vi "Read Image Delays.vi"(8 "error in (no error)":errorcluster, 11 "Header Contents in":refnum<class "Header Contents.lvclass">) -> (0 "error out":errorcluster, 2 "Image Delays":string[](array[string]), 3 "Header Contents out":refnum<class "Header Contents.lvclass">)   [LabVIEW 2018, in "Header Contents.lvclass"]
uses:
  Header Contents.lvclass
  Header Contents.lvclass/Header Contents.ctl
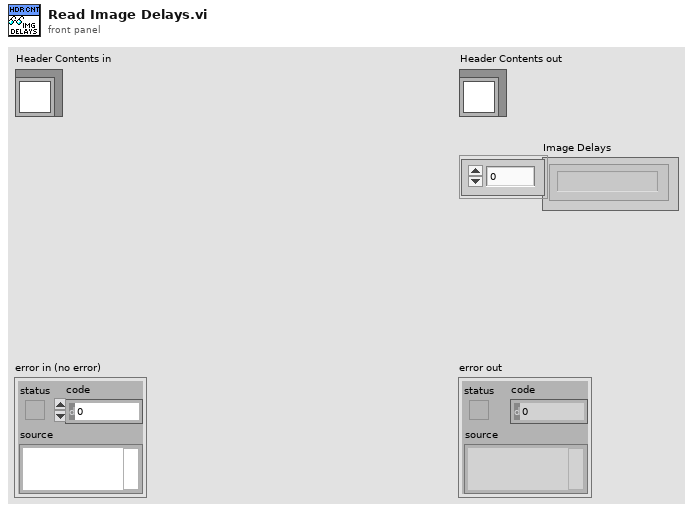
[diagram p1: front panel]
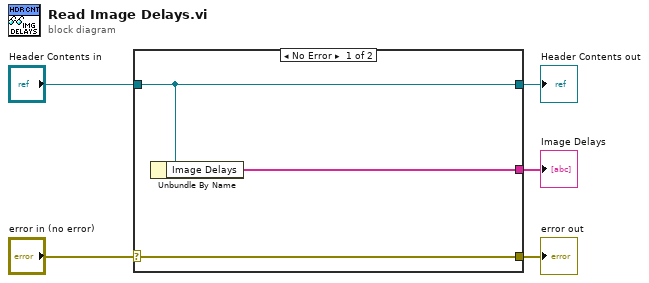
[diagram p0: block diagram]
diagram:
  n1 = case shown="No Error" "error in (no error)" {
    selector: "error in (no error)" -> [w8 w9]
    tunnel: [w8 w9] -> w4
    tunnel: [w7 w10] -> w2
    tunnel: "Header Contents in" -> [w7 w10]
    tunnel: [w6 _] -> w1
    frame No Error {
      n2 = Unbundle By Name(w7) -> ("Image Delays"=w6:string[])
    }
    frame Error {
    }
  }
  "error out" <- w4
  "Header Contents out" <- w2
  "Image Delays" <- w1
